vi "ScanAction.vi"(8 "error in (no error)":errorcluster caption="entrée d'erreur (pas d'erreur)", 9 "IndicePoint":i32, 10 "Dir":bool, 11 "Tools In":refnum<class "BNC845.lvclass"> caption="DNL_LabVIEW Object in") -> (0 "error out":errorcluster caption="sortie d'erreur", 2 "ScanParsOut":dbl[](array[numeric]), 3 "Tools Out":refnum<class "BNC845.lvclass"> caption="DNL_LabVIEW Object out")   [LabVIEW 2019, in "BNC845.lvclass"]
uses:
  BNC845.lvclass
  C:/Programmes Labview/LabScanV1A/DevicesClass/BaseDevice/BaseDevice.lvclass
  BNC845.lvclass/BNC845.ctl
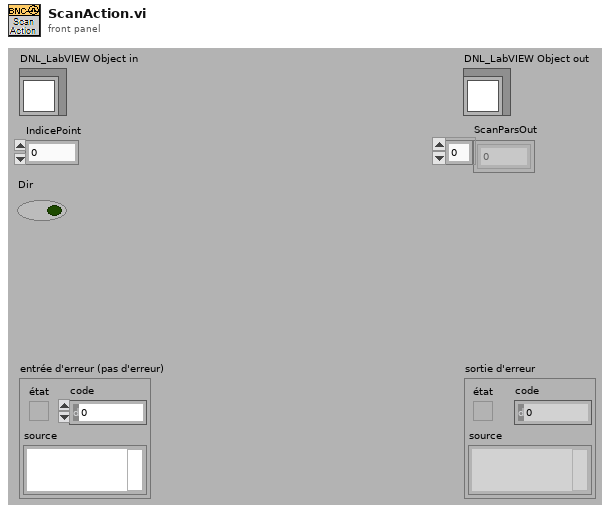
[diagram p1: front panel]
types:
  T1 = typedef "BNC845.lvclass/BNC845_Func.ctl" = enum16{"SetPower (dBm)", "SetFrequency (Hz)"}
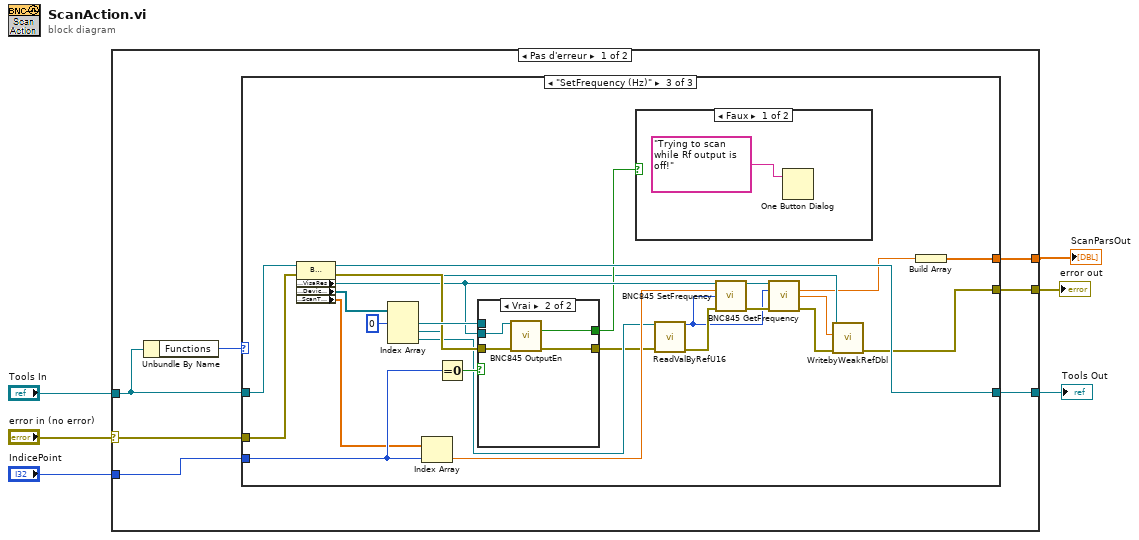
[diagram p0: block diagram]
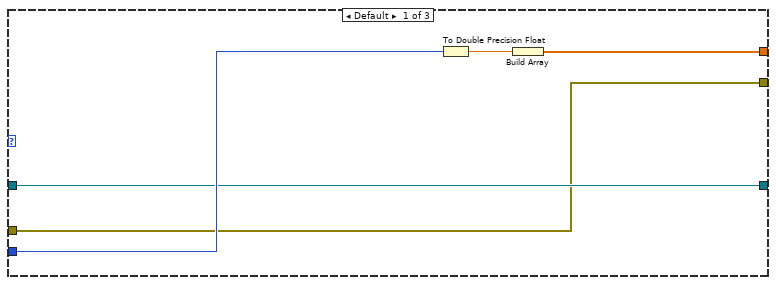
[diagram p2: hidden frame]
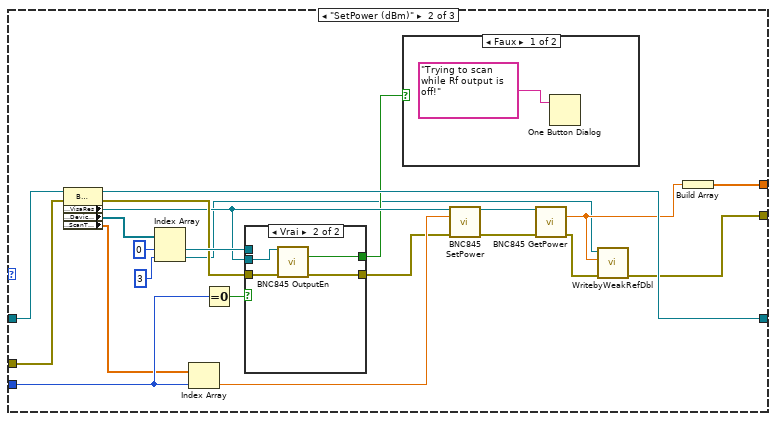
[diagram p3: hidden frame]
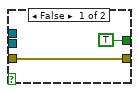
[diagram p5: hidden frame]
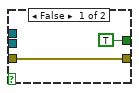
[diagram p7: hidden frame]
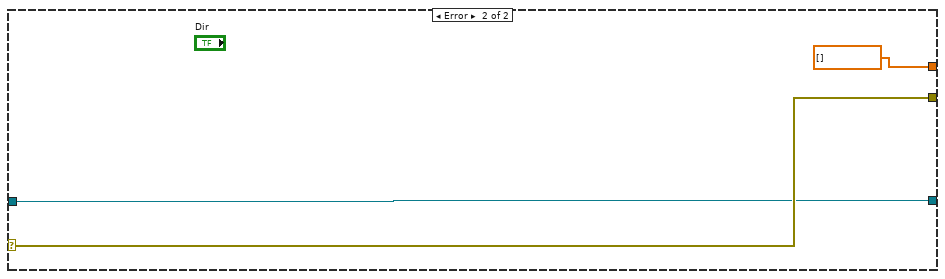
[diagram p8: hidden frame]
diagram:
  n1 = case shown="Pas d'erreur" "error in (no error)" {
    selector: "error in (no error)" -> [w10 w82]
    tunnel: "Tools In" -> [w11 w81]
    tunnel: [w9 dbl[] []] -> w1
    tunnel: [w8 w82] -> w4
    tunnel: [w7 w81] -> w3
    tunnel: "IndicePoint" -> [w12 _]
    frame No Error {
      n2 = Unbundle By Name(w11) -> ("Functions"=w13:T1)
      n3 = case shown="\"SetFrequency (Hz)\"" w13 {
        tunnel: [w14 w35 w67] -> w9
        tunnel: w12 -> [w18 w26 w60]
        tunnel: [w16 w34 w66] -> w7
        tunnel: w11 -> [w16 w31 w64]
        tunnel: w10 -> [w15 w38 w70]
        tunnel: [w15 w20 w56] -> w8
        frame Default {
          n4 = To Double Precision Float(number=w18) -> (double precision float=w17:dbl)
          n5 = Build Array(w17) -> (w14:dbl[])
        }
        frame "SetPower (dBm)" {
          n6 = property class="BNC845.lvclass"(reference=w31, error in=w38) -> (reference out=w34:refnum<class "BNC845.lvclass">, error out=w29:errorcluster, "Accessor:VisaRes"=w25:refnum<visa-resource-name>, "Accessor:DeviceCtrl"=w36:refnum<vi>[], "Accessor:ScanTable"=w19:dbl[])
          n7 = Index Array(array=w36, index #1=0 ("indice"), index #2=3 ("indice")) -> (element #1=w30:refnum<vi>, element #2=w21:refnum<vi>)
          n8 = Index Array(array=w19, index=w26) -> (element=w37:dbl)
          n9 = Equal To 0?(x=w26) -> (x = 0?=w27:bool)
          n10 = case shown="Vrai" w27 {
            tunnel: w30 -> [_ _]
            tunnel: w29 -> [w43 w46]
            tunnel: [w43 w45] -> w28
            tunnel: w25 -> [_ w47]
            tunnel: [TRUE ("Enabled") w44] -> w24
            frame False {
            }
            frame True {
              n11 = call <instrlib>:"BNC845 OutputEn.vi"("VISA Rsrc"=w47, "error in (no error)"=w46) -> ("Enabled"=w44:bool, "error out"=w45:errorcluster)  [unwired: 11 in, 1 out]
            }
          }
          n12 = case shown="Faux" w24 {
            frame False {
              n13 = One Button Dialog(message="Trying to scan while Rf output is off!") -> ()  [unwired: 1 in, 1 out]
            }
            frame True {
            }
          }
          n14 = call <instrlib>:"BNC845 SetPower.vi"("VISA Rsrc"=w25, "Power dBm"=w37, "error in (no error)"=w28) -> ("VISA Rsrc Out"=w39:refnum<visa-resource-name>, "error out"=w40:errorcluster)  [unwired: 11 in]
          n15 = call <instrlib>:"BNC845 GetPower.vi"("VISA Rsrc"=w39, "error in (no error)"=w40) -> ("Power (dBm)"=w22:dbl, "error out"=w23:errorcluster)  [unwired: 11 in, 1 out]
          n16 = call <userlib>:"WritebyWeakRefDbl.vi"("error in"=w23, "Valeur"=w22, "Control Ref"=w21) -> ("error out"=w20:errorcluster)  [unwired: 8 in]
          n17 = Build Array(w22) -> (w35:dbl[])
        }
        frame "SetFrequency (Hz)" {
          n18 = property class="BNC845.lvclass"(reference=w64, error in=w70) -> (reference out=w66:refnum<class "BNC845.lvclass">, error out=w62:errorcluster, "Accessor:VisaRes"=w59:refnum<visa-resource-name>, "Accessor:DeviceCtrl"=w68:refnum<vi>[], "Accessor:ScanTable"=w49:dbl[])
          n19 = Index Array(array=w68, index #1=0 ("indice")) -> (element #1=w63:refnum<vi>, element #2=w55:refnum<vi>, element #3=w54:refnum<vi>)  [unwired: 2 in]
          n20 = Index Array(array=w49, index=w60) -> (element=w69:dbl)
          n21 = Equal To 0?(x=w60) -> (x = 0?=w61:bool)
          n22 = case shown="Vrai" w61 {
            tunnel: w63 -> [_ _]
            tunnel: w62 -> [w75 w78]
            tunnel: [w75 w77] -> w53
            tunnel: w59 -> [_ w79]
            tunnel: [TRUE ("Enabled") w76] -> w58
            frame False {
            }
            frame True {
              n23 = call <instrlib>:"BNC845 OutputEn.vi"("VISA Rsrc"=w79, "error in (no error)"=w78) -> ("Enabled"=w76:bool, "error out"=w77:errorcluster)  [unwired: 11 in, 1 out]
            }
          }
          n24 = case shown="Faux" w58 {
            frame False {
              n25 = One Button Dialog(message="Trying to scan while Rf output is off!") -> ()  [unwired: 1 in, 1 out]
            }
            frame True {
            }
          }
          n26 = call <userlib>:"ReadValByRefU16.vi"("Control Ref"=w54, "error in"=w53) -> ("Valeur"=w51:u16, "error out"=w52:errorcluster)  [unwired: 12 in]
          n27 = call <instrlib>:"BNC845 SetFrequency.vi"("VISA Rsrc"=w59, "Frequency (Hz)"=w69, "FUnits"=w51, "error in (no error)"=w52) -> ("VISA Rsrc Out"=w71:refnum<visa-resource-name>, "error out"=w72:errorcluster)  [unwired: 10 in]
          n28 = call <instrlib>:"BNC845 GetFrequency.vi"("VISA Rsrc"=w71, "FUnits"=w51, "error in (no error)"=w72) -> ("Frequency (Hz)"=w48:dbl, "Frequency (Units)"=w50:dbl, "error out"=w57:errorcluster)  [unwired: 9 in, 1 out]
          n29 = call <userlib>:"WritebyWeakRefDbl.vi"("error in"=w57, "Valeur"=w50, "Control Ref"=w55) -> ("error out"=w56:errorcluster)  [unwired: 8 in]
          n30 = Build Array(w48) -> (w67:dbl[])
        }
      }
    }
    frame Error {
    }
  }
  "error out" <- w4
  "Tools Out" <- w3
  "ScanParsOut" <- w1
